vi "Measure_Voltage.vi"(8 "error in (no error)":errorcluster, 10 "Measure_Configuration":variant, 11 "NI-DMM in":refnum<class "NI-DCPower.lvclass">) -> (0 "error out":errorcluster, 2 "DC_Voltage":dbl, 3 "NI-DMM out":refnum<class "NI-DCPower.lvclass">)   [LabVIEW 2020, in "NI-DCPower.lvclass"]
uses:
  NI-DCPower.lvclass
  C:/Program Files/National Instruments/LabVIEW 2020/vi.lib/MeasurementLink/MeasurementLink Instrument/ISession Factory/ISession Factory.lvclass
  Typedefs/Configure_Parameters.ctl
  <vilib>/MeasurementLink/MeasurementLink Session Management V1/Session Reservation/Pin Type.ctl
  Typedefs/connection with session.ctl
  <vilib>/MeasurementLink/MeasurementLink Session Management V1/Session Reservation/Connection.ctl
  <instrlib>/niDCPower/nidcpower.llb/niDCPower Wait For Event - Event.ctl
  <instrlib>/niDCPower/nidcpower.llb/niDCPower Measurement Type.ctl
  ecdb0463-d15a-4b68-8fc7-7eeeceb900b2.vi
  <vilib>/MeasurementLink/MeasurementLink Session Management V1/Session Reservation/Get Connections Impl.vi
  NI-DCPower.lvclass/NI-DCPower.ctl
  <vilib>/MeasurementLink/MeasurementLink Session Management V1/Session Reservation/Session Reservation.lvclass
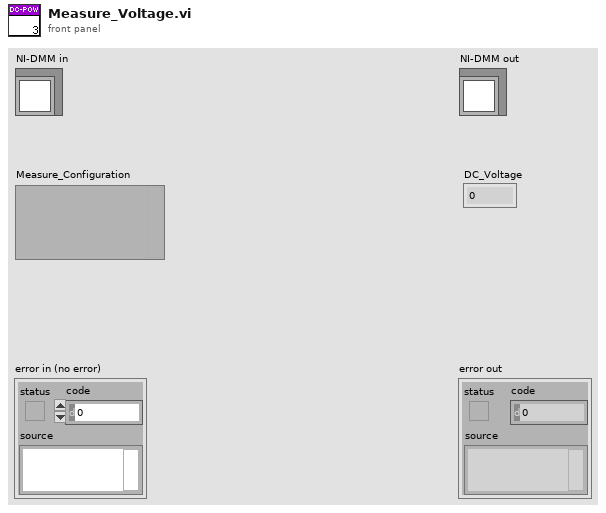
[diagram p1: front panel]
types:
  T1 = typedef "NI-DCPower.lvclass/connection with session.ctl" = cluster{"connection":T2, "session":refnum<k15>}
  T2 = typedef "MeasurementLink Session Management V1.lvlib/Session Reservation.lvclass/Connection.ctl" = cluster{"pin or relay name":string, "site":i32, "instrument type id":string, "channel":string}
  T3 = typedef "MeasurementLink Session Management V1.lvlib/Session Reservation.lvclass/Pin Type.ctl" = enum16{"DUT and System Pins", "System Pins"}
  T4 = typedef "NI-DCPower.lvclass/Configure_Parameters.ctl" = cluster{"pin name":string[], "Range":dbl, "Measurement Type":enum32{"DC Volts", "AC Volts", "DC Current", "AC Current", "2-wire Resistance", "4-wire Resistance", "Diode", "Frequency", "Period", "AC Volts DC Coupled", "Capacitance", "Inductance", "Temperature"}, "Resolution in Digits":enum32{"3 1/2", "4 1/2", "5 1/2", "6 1/2", "7 1/2"}}
  T5 = typedef "niDCPower Measurement Type.ctl" = i32
  T6 = typedef "niDCPower Wait For Event - Event.ctl" = i32
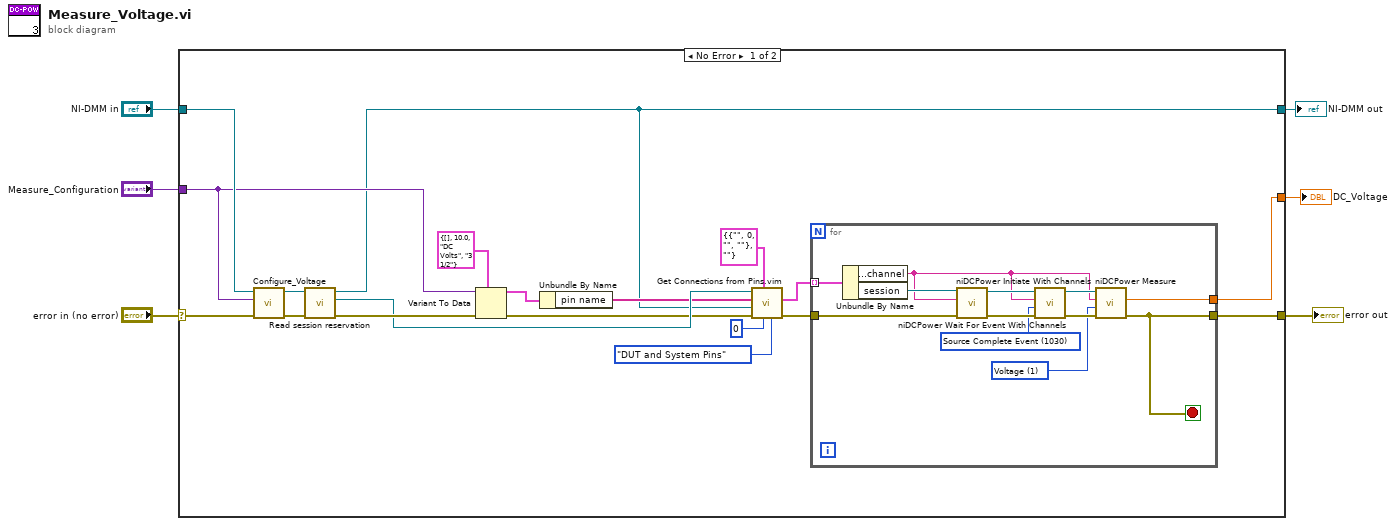
[diagram p0: block diagram]
diagram:
  n1 = case shown="No Error" "error in (no error)" {
    selector: "error in (no error)" -> [w25 w38]
    tunnel: "NI-DMM in" -> [w24 w39]
    tunnel: [w23 w38] -> w4
    tunnel: [w22 _] -> w3
    tunnel: "Measure_Configuration" -> [w20 _]
    tunnel: [w10 w39] -> w1
    frame No Error {
      n2 = call-dynamic "Configure_Voltage.vi"("error in (no error)"=w25, "DC_Voltage_Configuration"=w20, "NI-DMM in"=w24) -> ("error out"=w19:errorcluster, "NI-DMM out"=w16:refnum<class "NI-DCPower.lvclass">)  [unwired: 7 in]
      n3 = call-dynamic "Read session reservation.vi"("error in (no error)"=w19, "Abstract_Instrument in"=w16) -> ("error out"=w17:errorcluster, "Session Reservation.lvclass"=w15:refnum<class "Session Reservation.lvclass">, "Abstract_Instrument out"=w10:refnum<class "NI-DCPower.lvclass">)  [unwired: 7 in]
      n4 = Variant To Data(error in=w17, type=T4 {"pin name"=[], "Range"=10.0, "Measurement Type"=enum."DC Volts", "Resolution in Digits"=enum."3 1/2"}, Variant=w20) -> (data=w18:T4, error out=w14:errorcluster)
      n5 = Unbundle By Name(w18) -> ("pin name"=w11:string[])
      n6 = call "Get Connections from Pins.vim"("pin type"=Pin_Type."DUT and System Pins", "site"=0, "connection type"=T1 {"connection"={"pin or relay name"="", "site"=0, "instrument type id"="", "channel"=""}, "session"=""} ("connection with session"), "error in"=w14, "session factory"=w10, "pin or relay names"=w11, "session reservation in"=w15) -> ("error out"=w13:errorcluster, "connections"=w12:T1[])  [unwired: 2 in, 1 out]
      n7 = for {
        tunnel: [w28] -> w22
        tunnel: w12 -> [w33] mode=indexing
        tunnel: w13 -> [w34]
        tunnel: [w29] -> w23
        stop <- w29 stop-if-true
        w26 = T5 1 items=["Current", "Voltage"] ("measurement type")
        w35 = T6 1030 items=["Source Complete Event"=1030, "Measure Complete Event"=1031, "Sequence Iteration Complete Event"=1032, "Sequence Engine Done Event"=1033, "Pulse Complete Event"=1051, "Ready For Pulse Trigger Event"=1052] ("event")
        n8 = Unbundle By Name(w33) -> ("connection.channel"=w27:string, "session"=w32:refnum<k15>)
        n9 = call <instrlib>:"niDCPower Initiate With Channels.vi"("error in (no error)"=w34, "channel name"=w27, "instrument handle"=w32) -> ("error out"=w36:errorcluster, "instrument handle out"=w37:refnum<k15>)  [unwired: 7 in]
        n10 = call <instrlib>:"niDCPower Wait For Event With Channels.vi"("error in (no error)"=w36, "event"=w35, "channel name"=w27, "instrument handle"=w37) -> ("error out"=w31:errorcluster, "instrument handle out"=w30:refnum<k15>)  [unwired: 6 in]
        n11 = call <instrlib>:"niDCPower Measure.vi"("error in (no error)"=w31, "measurement type"=w26, "channel name"=w27, "instrument handle"=w30) -> ("error out"=w29:errorcluster, "measurement"=w28:dbl)  [unwired: 5 in, 1 out]
      }
    }
    frame Error {
    }
  }
  "error out" <- w4
  "NI-DMM out" <- w1
  "DC_Voltage" <- w3
